vi "estiDof.vi"() -> ()   [LabVIEW 2016]
uses:
  OptCtrl/OptCtrl.lvclass
  OptStateEsti/OptStateEsti.lvclass
  StrictDef/FilterType.ctl
  StrictDef/InstName.ctl
  StrictDef/DofGroup.ctl
panel:
  out "M2 Bending mode":dbl[](array[numeric])
  out "M1M3 Bending mode":dbl[](array[numeric])
  out "Cam Position":dbl[](array[numeric])
  out "M2 Position":dbl[](array[numeric])
  in  "DOF Data":path=path "/home/ttsai/Documents/stash/ts_tcs_ofc/testData/sim6_iter1_pert.txt"
  out "DOF Array":dbl[](array[numeric])
  out "State in DOF":dbl[](array[numeric])
  in  "Configuration":T2={"Config Dir"=path "/home/ttsai/Documents/stash/ts_tcs_ofc/configData", "Config File Name"="optiPSSN_x00.ctrl", "Inst Name"=enum."lsst", "State 0 File Name"="state0inDof.txt", "Weighting File Name"="imgQualWgt.txt", "PSSN Alpha File Name"="pssn_alpha.txt", "Authority Files"={"Rigid Body Stroke File"="rbStroke.txt", "M1M3 Subsystem"={"Mirror"="M1M3", "Actuatro Force File"="M1M3_1um_156_force.txt"}, "M2 Subsystem"={"Mirror"="M2", "Actuatro Force File"="M2_1um_force.DAT"}, "Num of Bending Mode"=20}}
  in  "Filter Type":T3
  out "uk Array":dbl[](array[numeric])
  out "State in DOF 0":dbl[](array[numeric])
  out "F Matrix":dbl[][](array[numeric])
  in  "OptStateEsti in":refnum<class "OptStateEsti.lvclass">
  out "Range of DOF":dbl[](array[numeric])
  out "Authority":dbl[](array[numeric])
  in  "Gain":dbl=1.0
  in  "OptCtrl in":refnum<class "OptCtrl.lvclass">
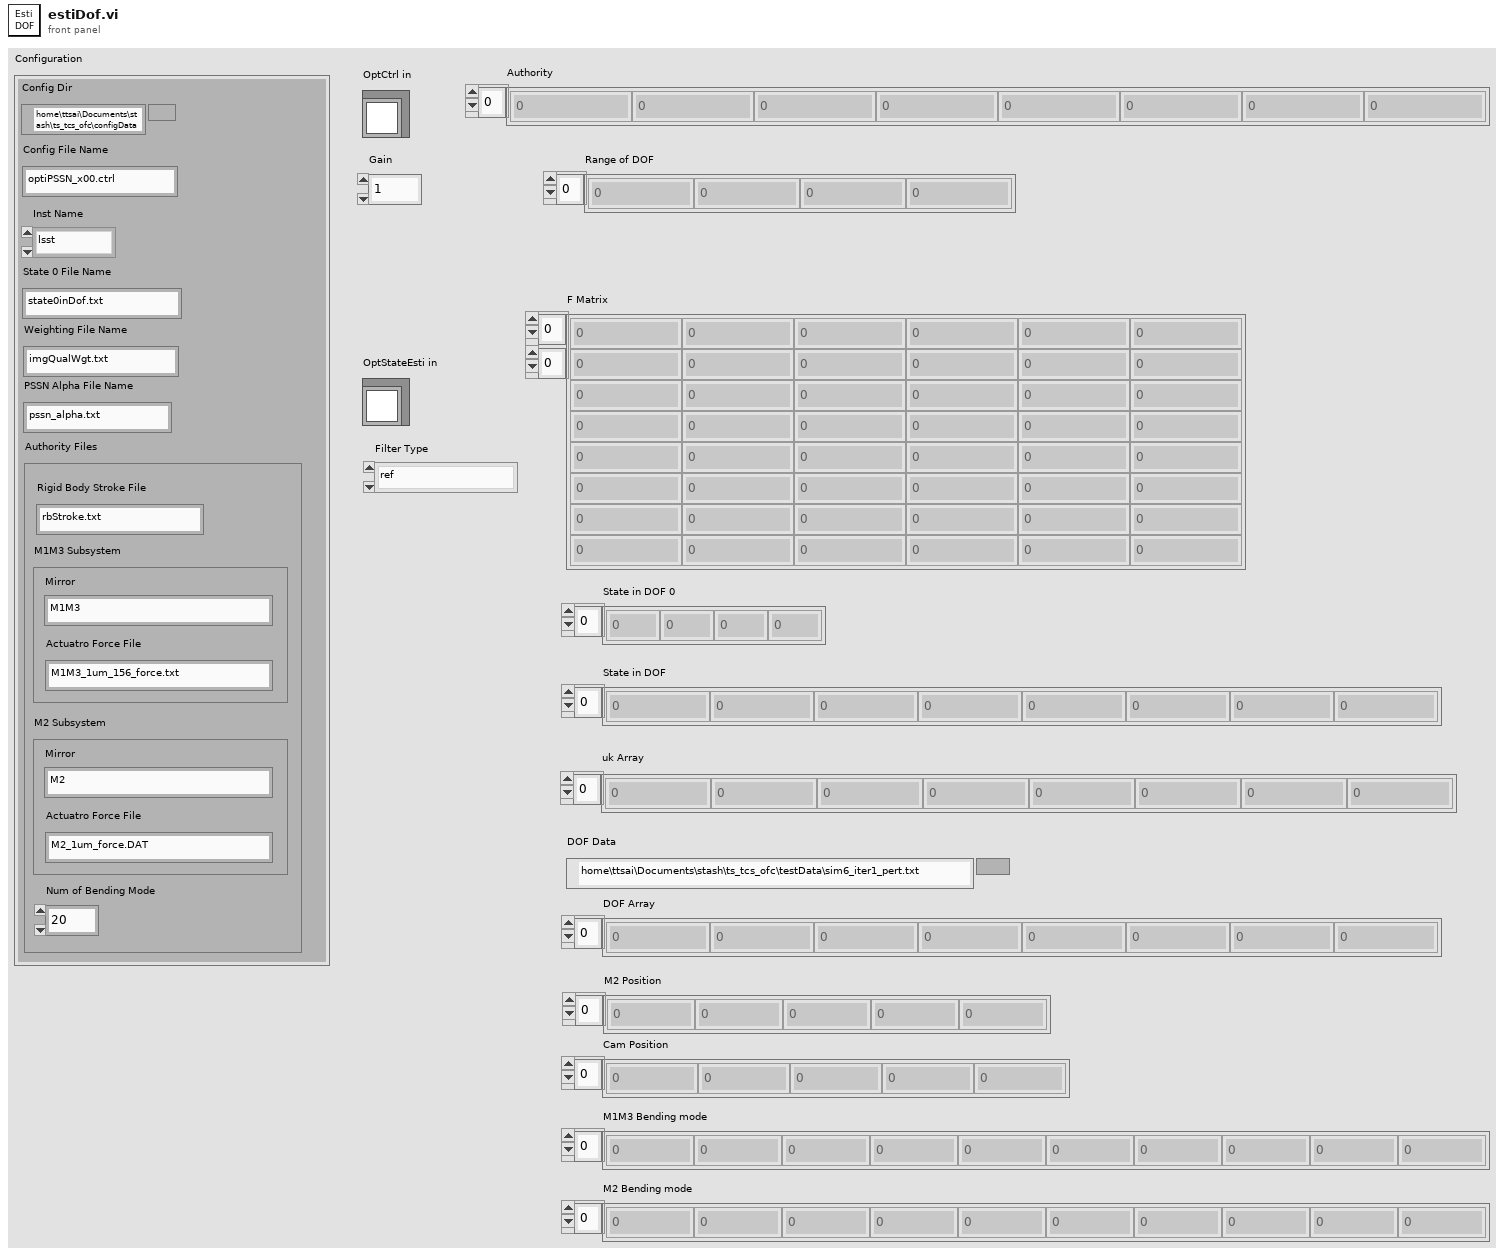
[diagram p1: front panel]
types:
  T1 = typedef "InstName.ctl" = enum16{"lsst", "comcam"}
  T2 = cluster{"Config Dir":path, "Config File Name":string, "Inst Name":T1, "State 0 File Name":string, "Weighting File Name":string, "PSSN Alpha File Name":string, "Authority Files":cluster{"Rigid Body Stroke File":string, "M1M3 Subsystem":cluster{"Mirror":string, "Actuatro Force File":string}, "M2 Subsystem":cluster{"Mirror":string, "Actuatro Force File":string}, "Num of Bending Mode":i32}}
  T3 = typedef "FilterType.ctl" = enum16{"ref", "u", "g", "r", "i", "z", "y"}
  T4 = typedef "DofGroup.ctl" = enum16{"M2 Hex Pos", "Cam Hex Pos", "M1M3 Bend", "M2 Bend"}
  T5 = enum16{"M2 Hex Pos", "Cam Hex Pos", "M1M3 Bend", "M2 Bend"}
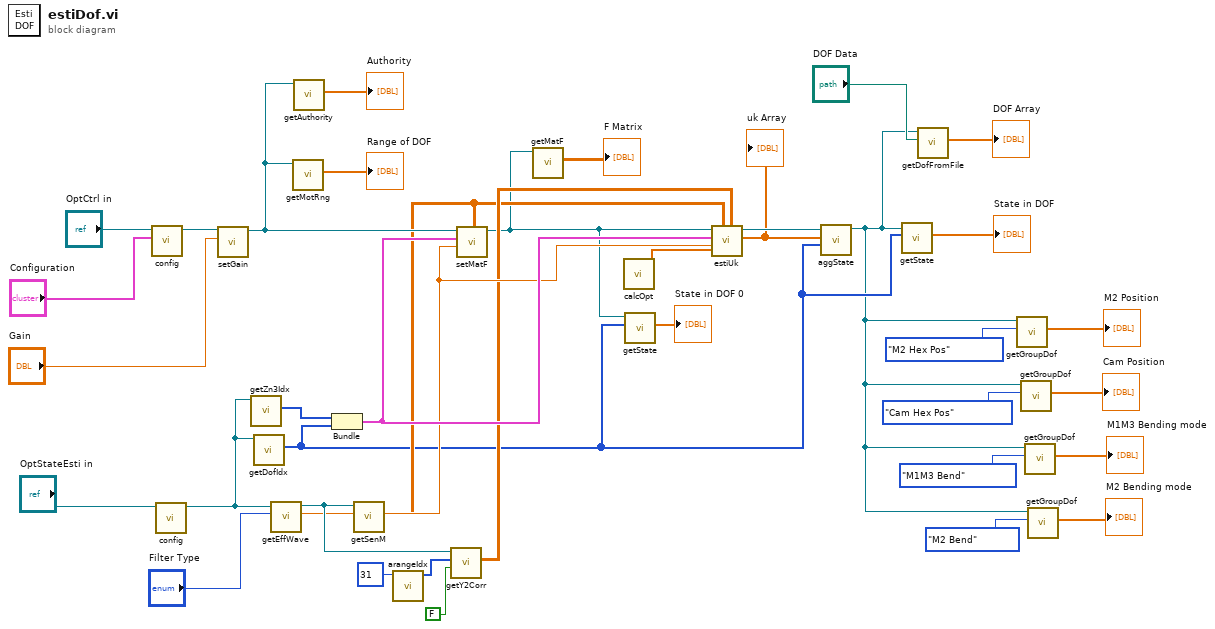
[diagram p0: block diagram]
diagram:
  n1 = call "config.vi"("Configuration"="Configuration", "OptCtrl in"="OptCtrl in") -> ("OptCtrl out"=w29:refnum<class "OptCtrl.lvclass">)  [unwired: 8 in, 1 out]
  n2 = call "config.vi"("OptStateEsti in"="OptStateEsti in") -> ("OptStateEsti out"=w33:refnum<class "OptStateEsti.lvclass">)  [unwired: 9 in, 1 out]
  n3 = call "setGain.vi"("Gain"="Gain", "OptCtrl in"=w29) -> ("OptCtrl out"=w21:refnum<class "OptCtrl.lvclass">)  [unwired: 8 in, 1 out]
  n4 = call "getZn3Idx.vi"("OptStateEsti in"=w33) -> ("zn3Idx"=w27:i32[])  [unwired: 8 in, 2 out]
  n5 = call "getDofIdx.vi"("OptStateEsti in"=w33) -> ("dofIdx"=w13:i32[])  [unwired: 8 in, 2 out]
  n6 = call "getEffWave.vi"("Filter Type"="Filter Type", "OptStateEsti in"=w33) -> ("Effective Wavelength  (um)"=w24:dbl, "OptStateEsti out"=w36:refnum<class "OptStateEsti.lvclass">)  [unwired: 7 in, 1 out]
  n7 = call "getMotRng.vi"("OptCtrl in"=w21) -> ("Range of DOF"=→"Range of DOF":dbl[])  [unwired: 8 in, 2 out]
  n8 = call "getAuthority.vi"("OptCtrl in"=w21) -> ("Authority"=→"Authority":dbl[])  [unwired: 8 in, 2 out]
  n9 = Bundle("zn3Idx"=w27, "dofIdx"=w13) -> (w25:cluster{"zn3Idx":i32[], "dofIdx":i32[]})  [unwired: 1 in]
  n10 = call "getSenM.vi"("OptStateEsti in"=w36) -> ("Sen M"=w18:dbl[][][])  [unwired: 8 in, 2 out]
  n11 = call "arangeIdx.vi"("Number"=31) -> ("Idx Array"=w35:i32[])  [unwired: 10 in]
  n12 = call "getY2Corr.vi"("In nx1 Row"=FALSE, "Field Idx"=w35, "OptStateEsti in"=w36) -> ("y2c Array"=w22:dbl[][])  [unwired: 6 in, 2 out]
  n13 = call "setMatF.vi"("Sen M"=w18, "Effective Wavelength"=w24, "Idx Group"=w25, "OptCtrl in"=w21) -> ("OptCtrl out"=w17:refnum<class "OptCtrl.lvclass">)  [unwired: 6 in, 1 out]
  n14 = call "getMatF.vi"("OptCtrl in"=w17) -> ("F Matrix"=→"F Matrix":dbl[][])  [unwired: 8 in, 2 out]
  n15 = call "calcOpt.vi"() -> ("Optical State"=w23:dbl[])  [unwired: 11 in]
  n16 = call "getState.vi"("dofIdx"=w13, "OptCtrl in"=w17) -> ("State in DOF"=→"State in DOF 0":dbl[])  [unwired: 7 in, 2 out]
  n17 = call "estiUk.vi"("y2 Matrix"=w22, "Optical State"=w23, "Sen M"=w18, "Effective Wavelength"=w24, "Idx Group"=w25, "OptCtrl in"=w17) -> ("uk Array"=w14:dbl[], "OptCtrl out"=w15:refnum<class "OptCtrl.lvclass">)  [unwired: 3 in, 1 out]
  "uk Array" <- w14
  n18 = call "aggState.vi"("dofIdx"=w13, "State in DOF"=w14, "OptCtrl in"=w15) -> ("OptCtrl out"=w4:refnum<class "OptCtrl.lvclass">)  [unwired: 7 in, 1 out]
  n19 = call "getState.vi"("dofIdx"=w13, "OptCtrl in"=w4) -> ("State in DOF"=→"State in DOF":dbl[])  [unwired: 7 in, 2 out]
  n20 = call "getDofFromFile.vi"("DOF Data"="DOF Data", "OptCtrl in"=w4) -> ("DOF Array"=→"DOF Array":dbl[])  [unwired: 7 in, 2 out]
  n21 = call "getGroupDof.vi"("DOF Group"=DofGroup."M2 Hex Pos", "OptCtrl in"=w4) -> ("DOF"=→"M2 Position":dbl[])  [unwired: 7 in, 2 out]
  n22 = call "getGroupDof.vi"("DOF Group"=T5."Cam Hex Pos", "OptCtrl in"=w4) -> ("DOF"=→"Cam Position":dbl[])  [unwired: 7 in, 2 out]
  n23 = call "getGroupDof.vi"("DOF Group"=T5."M1M3 Bend", "OptCtrl in"=w4) -> ("DOF"=→"M1M3 Bending mode":dbl[])  [unwired: 7 in, 2 out]
  n24 = call "getGroupDof.vi"("DOF Group"=T5."M2 Bend", "OptCtrl in"=w4) -> ("DOF"=→"M2 Bending mode":dbl[])  [unwired: 7 in, 2 out]
